vi "Init_serial.vi"(11 "Serial Name (port)":string) -> (0 "error out":errorcluster, 3 "Python out":cluster{"Python":refnum<k35>, "py file":path})   [LabVIEW 2020]
panel:
  out "return value":string
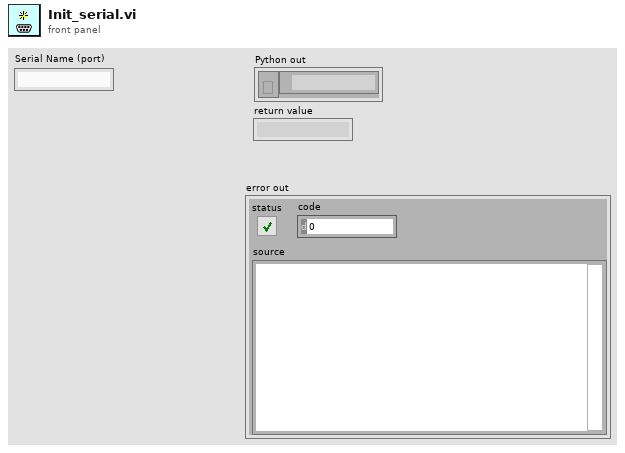
[diagram p1: front panel]
types:
  T1 = cluster{"session out":refnum<k35>, "appended path":path}
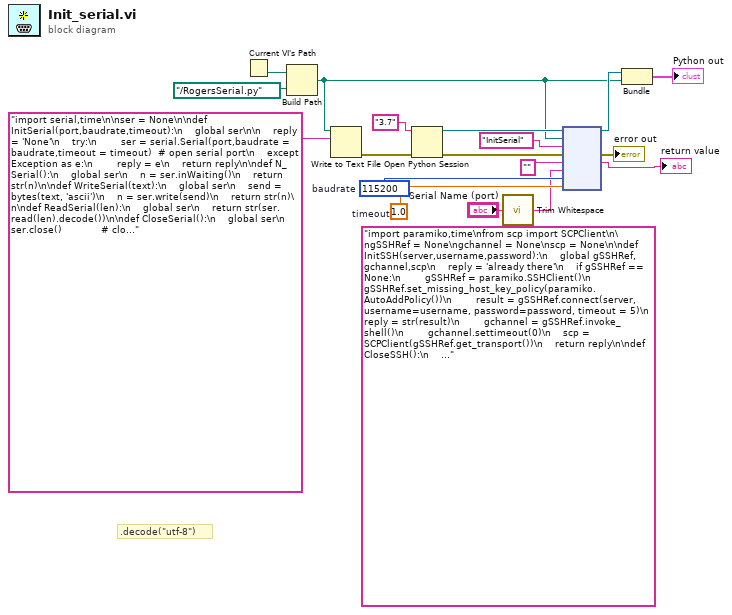
[diagram p0: block diagram]
diagram:
  w5 = 1.0  # timeout
  w4 = 115200  # baudrate
  (unwired) "import paramiko,time\nfrom scp import SCPClient\n\ngSSHRef = None\ngchannel = None\nscp = None\n\ndef InitSSH(server,username,password):\n    global gSSHRef, gchannel,scp\n    reply = 'already there'\n    if gSSHRef == None:\n        gSSHRef = paramiko.SSHClient()\n        gSSHRef.set_missing_host_key_policy(paramiko.AutoAddPolicy())\n        result = gSSHRef.connect(server, username=username, password=password, timeout = 5)\n        reply = str(result)\n        gchannel = gSSHRef.invoke_shell()\n        gchannel.settimeout(0)\n    scp = SCPClient(gSSHRef.get_transport())\n    return reply\n\ndef CloseSSH():\n    if gchannel != None:\n        gchannel.close()\n    if gSSHRef != None:\n        gSSHRef.close()\n    if scp != None:\n        scp.close()\n    return('done')\n\ndef WriteSSH(string):\n    reply = 'no reference'\n    if gSSHRef != None:\n        reply = 'no file'\n        if gchannel != None:\n            size = gchannel.send(string.encode())\n            reply = str(size)\n    return reply\n\ndef ReadSSH():\n    reply = 'no reference'\n    if gSSHRef != None:\n        reply = 'no file'\n        if gchannel != None:\n            reply = ''\n            if gchannel.recv_ready():\n                reply = gchannel.recv(9999).decode()\n\n    return(reply)\n\ndef WriteWaitReadSSH(string,char,timeout=10000):\n     reply = ''\n     WriteSSH(string)\n     n = int(timeout/10)\n     for i in range(n):\n         ans = ReadSSH()\n         if ans.find(char) >= 0:\n             print(ans)\n             return reply + ans\n         reply = reply + ans\n         time.sleep(0.01)\n     return reply\n\ndef scp_get(name):\n     try:\n          scp.get(name)\n          return 'get succeeded\\n'\n     except Exception as e:\n          return  'scp.get('+name+')\\n' +str(e)\n\ndef scp_put(source, dest):\n     try:\n          scp.put(source, dest)\n          return 'scp.put('+source+','+dest+')\\n' +'put succeeded\\n'\n     except Exception as e:\n          return str(e)\n\ndef scp_put_all(source, dest):\n     try:\n          scp.put(source, recursive = True, remote_path = dest)\n          return 'put succeeded\\n'\n     except Exception as e:\n          return str(e)\n" ("name or relative path")
  # ".decode(\"utf-8\")"
  n1 = Current VI's Path() -> (path=w8:path)
  n2 = Build Path(base path=w8, name or relative path=path "../RogersSerial.py" ("base path")) -> (appended path=w12:path)
  n3 = Write to Text File(file (use dialog)=w12, text="import serial,time\n\nser = None\n\ndef InitSerial(port,baudrate,timeout):\n    global ser\n\n    reply = 'None'\n    try:\n        ser = serial.Serial(port,baudrate = baudrate,timeout = timeout)  # open serial port\n    except Exception as e:\n        reply = e\n    return reply\n\ndef N_Serial():\n    global ser\n    n = ser.inWaiting()\n    return str(n)\n\ndef WriteSerial(text):\n    global ser\n    send = bytes(text, 'ascii')\n    n = ser.write(send)\n    return str(n)\n\ndef ReadSerial(len):\n    global ser\n    return str(ser.read(len).decode())\n\ndef CloseSerial():\n    global ser\n    ser.close()             # close port" ("name or relative path")) -> (error out=w18:errorcluster)  [unwired: 2 in, 2 out]
  n4 = Open Python Session(python version="3.7" ("Python version"), 3:w18) -> (session out=w13:refnum<k35>, error out=w10:errorcluster)  [unwired: 1 in]
  n5 = call <vilib>:"Trim Whitespace.vi"("string"="Serial Name (port)") -> ("trimmed string"=w3:string)  [unwired: 1 in]
  n6 = node(w13, w12, "InitSerial" ("function name"), w10, "", w3, w4, w5) -> (w15:refnum<k35>, →"error out":errorcluster, →"return value":string)  [unwired: 3 in, 2 out]
  n7 = Bundle("session out"=w15, "appended path"=w12) -> (→"Python out":T1)  [unwired: 1 in]
